vi "DAC_set_use_buses.vi"(1 "FPGA Ref":T1, 2 "Use FPGA?":bool, 3 "Inst_array":T2(array[cluster])) -> (0 "FPGA VI Reference Out":T1)   [LabVIEW 2013]
uses:
  fpga-bitfile-ref.ctl
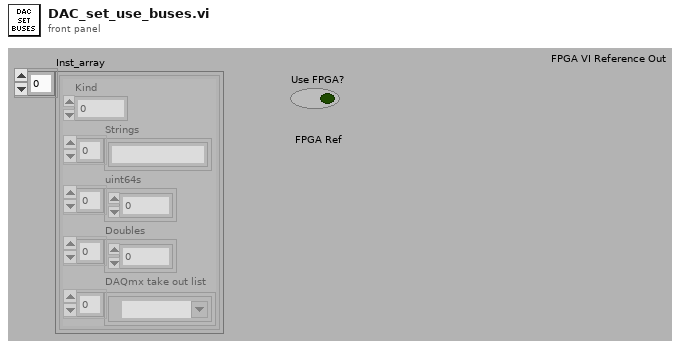
[diagram p1: front panel]
types:
  T1 = typedef "fpga-bitfile-ref.ctl" = refnum<k20>
  T2 = cluster{"Kind":u16, "Strings":string[], "uint64s":u64[], "Doubles":dbl[], "DAQmx take out list":refnum<k21>[]}[]
  T3 = enum8{"start movement", "buses to use", "delay", "value"}
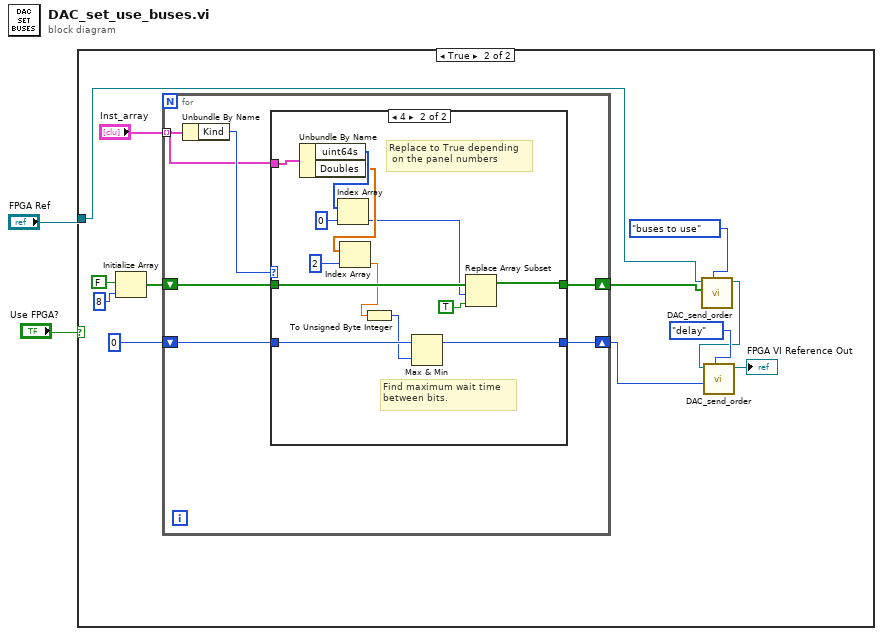
[diagram p0: block diagram]
diagram:
  n1 = case shown="True" "Use FPGA?" {
    tunnel: "FPGA Ref" -> [_ w8]
    frame False {
    }
    frame True {
      n2 = Initialize Array(FALSE, 8) -> (w11:bool[])
      n3 = for {
        tunnel: "Inst_array" -> [w19] mode=indexing
        shift-right: [w17] -> w9
        shift-left: w11 -> [w18]
        shift-right: [w15] -> w7
        shift-left: u8 0 -> [w16]
        n4 = Unbundle By Name(w19) -> ("Kind"=w20:u16)
        n5 = case shown="4" w20 {
          tunnel: w19 -> [_ w35]
          tunnel: w18 -> [w22 w30]
          tunnel: [w22 w23] -> w17
          tunnel: w16 -> [w21 w27]
          tunnel: [w21 w24] -> w15
          frame 0, Default {
          }
          frame 4 {
            # "Find maximum wait time\nbetween bits."
            # "Replace to True depending\n on the panel numbers"
            n6 = Unbundle By Name(w35) -> ("uint64s"=w34:u64[], "Doubles"=w33:dbl[])
            n7 = Index Array(array=w34, index=0) -> (element=w28:u64)
            n8 = Index Array(array=w33, index=2) -> (element=w25:dbl)
            n9 = To Unsigned Byte Integer(number=w25) -> (unsigned 8bit integer=w26:u8)
            n10 = Max & Min(x=w27, y=w26) -> (max(x,y)=w24:u8)  [unwired: 1 out]
            n11 = Replace Array Subset(array=w30, new element=TRUE, index=w28) -> (w23:bool[])
          }
        }
      }
      n12 = call "DAC_send_order.vi"("order"=T3."buses to use", "buses to use"=w9, "FPGA VI Reference In"=w8) -> ("FPGA VI Reference Out"=w5:T1)  [unwired: 4 in, 4 out]
      n13 = call "DAC_send_order.vi"("order"=T3."delay", "delay between steps (ms)"=w7, "FPGA VI Reference In"=w5) -> ("FPGA VI Reference Out"=→"FPGA VI Reference Out":T1)  [unwired: 4 in, 4 out]
    }
  }
